vi "cross_talk).vi"(9 "Array":u8[](array[numeric]), 10 "Rising Index 2":i32[](array[numeric]), 11 "Rising Index":i32[](array[numeric])) -> (2 "x/y 2":dbl, 3 "x/y":dbl)   [LabVIEW 2012]
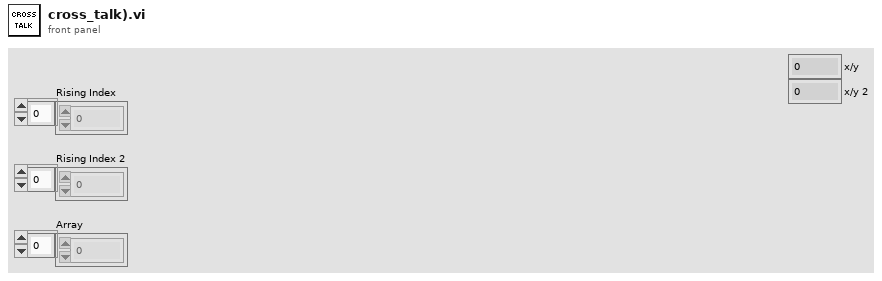
[diagram p1: front panel]
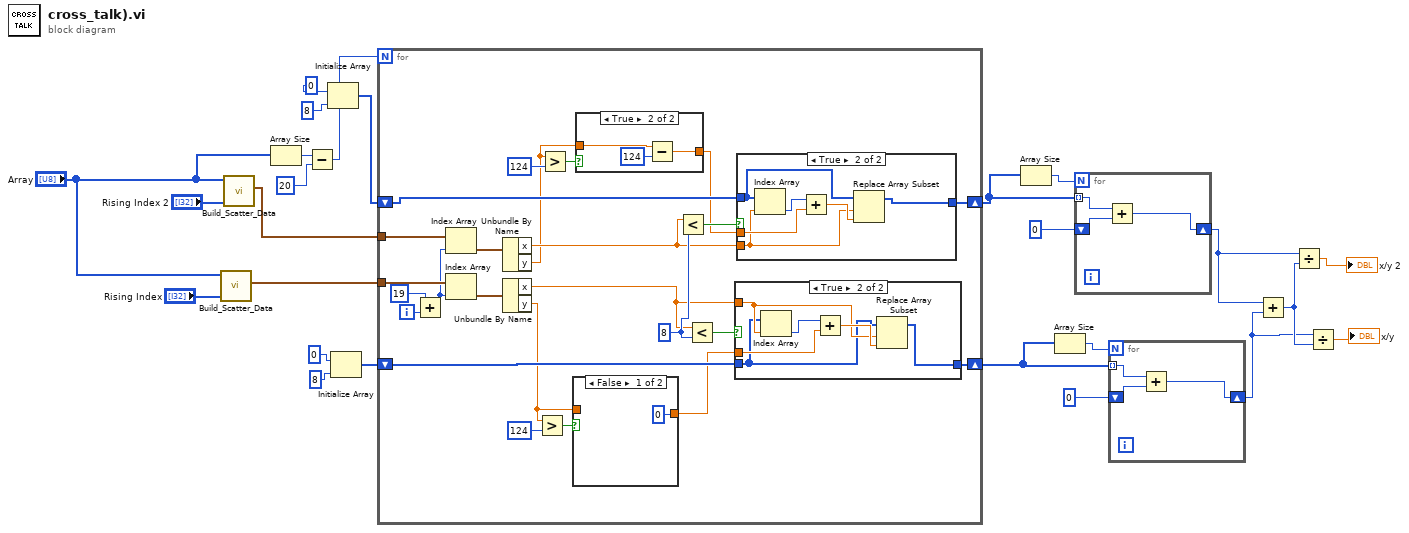
[diagram p0: block diagram]
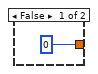
[diagram p2: hidden frame]
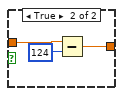
[diagram p3: hidden frame]
diagram:
  n1 = call "Build_Scatter_Data.vi"("Rising Index"="Rising Index", "PMT (AI 0)"="Array") -> ("data"=w18:cluster{"x":dbl, "y":dbl}[])  [unwired: 9 in]
  n2 = call "Build_Scatter_Data.vi"("Rising Index"="Rising Index 2", "PMT (AI 0)"="Array") -> ("data"=w19:cluster{"x":dbl, "y":dbl}[])  [unwired: 9 in]
  n3 = Array Size(array="Array") -> (size(s)=w22:i32)
  n4 = Subtract(x=w22, y=20) -> (x-y=w21:i32)
  n5 = Initialize Array(0, 8) -> (w12:i32[])
  n6 = Initialize Array(0, 8) -> (w16:i32[])
  n7 = for {
    N: w21 -> [_]
    tunnel: w19 -> [w47]
    tunnel: w18 -> [w46]
    shift-right: [w37] -> w6
    shift-left: w16 -> [w39]
    shift-right: [w34] -> w10
    shift-left: w12 -> [w36]
    i -> [w49]
    w40 = 8
    n8 = Add(x=19, y=w49) -> (x+y=w45:i32)
    n9 = Index Array(array=w47, index=w45) -> (element=w44:cluster{"x":dbl, "y":dbl})
    n10 = Index Array(array=w46, index=w45) -> (element=w43:cluster{"x":dbl, "y":dbl})
    n11 = Unbundle By Name(w44) -> ("x"=w35:dbl, "y"=w27:dbl)
    n12 = Unbundle By Name(w43) -> ("x"=w38:dbl, "y"=w30:dbl)
    n13 = Greater?(x=w30, y=124) -> (0:w33:bool)
    n14 = Greater?(x=w27, y=124) -> (0:w29:bool)
    n15 = case shown="False" w33 {
      tunnel: [0 w56] -> w31
      tunnel: w30 -> [_ w55]
      frame False {
      }
      frame True {
        n16 = Subtract(x=w55, y=124) -> (x-y=w56:dbl)
      }
    }
    n17 = case shown="True" w29 {
      tunnel: [0 w52] -> w26
      tunnel: w27 -> [_ w51]
      frame False {
      }
      frame True {
        n18 = Subtract(x=w51, y=124) -> (x-y=w52:dbl)
      }
    }
    n19 = Less?(x=w35, y=w40) -> (x < y?=w42:bool)
    n20 = Less?(x=w38, y=w40) -> (x < y?=w41:bool)
    n21 = case shown="True" w41 {
      tunnel: w39 -> [w58 w60]
      tunnel: w38 -> [_ w62]
      tunnel: w31 -> [_ w64]
      tunnel: [w58 w59] -> w37
      frame False {
      }
      frame True {
        n22 = Index Array(array=w60, index=w62) -> (element=w61:i32)
        n23 = Add(x=w61, y=w64) -> (x+y=w63:dbl)
        n24 = Replace Array Subset(array=w60, new element=w63, index=w62) -> (w59:i32[])
      }
    }
    n25 = case shown="True" w42 {
      tunnel: w36 -> [w65 w71]
      tunnel: w26 -> [_ w70]
      tunnel: w35 -> [_ w67]
      tunnel: [w65 w66] -> w34
      frame False {
      }
      frame True {
        n26 = Index Array(array=w71, index=w67) -> (element=w69:i32)
        n27 = Add(x=w69, y=w70) -> (x+y=w68:dbl)
        n28 = Replace Array Subset(array=w71, new element=w68, index=w67) -> (w66:i32[])
      }
    }
  }
  n29 = Array Size(array=w10) -> (size(s)=w11:i32)
  n30 = Array Size(array=w6) -> (size(s)=w8:i32)
  n31 = for {
    N: w11 -> [_]
    tunnel: w10 -> [w74] mode=indexing
    shift-right: [w72] -> w4
    shift-left: 0 -> [w73]
    n32 = Add(x=w74, y=w73) -> (x+y=w72:i32)
  }
  n33 = for {
    N: w8 -> [_]
    tunnel: w6 -> [w77] mode=indexing
    shift-right: [w75] -> w3
    shift-left: 0 -> [w76]
    n34 = Add(x=w77, y=w76) -> (x+y=w75:i32)
  }
  n35 = Add(x=w4, y=w3) -> (x+y=w5:i32)
  n36 = Divide(x=w4, y=w5) -> (x/y=→"x/y 2":dbl)
  n37 = Divide(x=w3, y=w5) -> (x/y=→"x/y":dbl)
